vi "SimplifiedCounter.vi"() -> ()   [LabVIEW 2020]
uses:
  <vilib>/Platform/TimedLoop/XDataNode/timing_clust.ctl
  <vilib>/Platform/TimedLoop/XDataNode/nitl_modes.ctl
  <vilib>/Platform/TimedLoop/XDataNode/wakeup.ctl
  <vilib>/rvi/Emulation/niFpgaGetClockAttributes.vi
  <vilib>/rvi/Emulation/niFpgaSctlEmulationGetInTimedLoop.vi
  <vilib>/rvi/Emulation/niFpgaEmulationReportErrorSimple.vi
  <vilib>/rvi/Emulation/niFpgaCriticalErrorInLSC.vi
  <vilib>/rvi/eio/common/nirviEmuTemplateMethod_errors.vi
  <vilib>/rvi/Emulation/niFpgaProcessEmulError.vi
  <vilib>/Platform/TimedLoop/XDataNode/XDataNode.xnode
  <vilib>/eio/EIONode/EIONode.xnode
  <vilib>/Platform/TimedLoop/XDataNode/XDNodeRunTimeDep.lvlib
panel:
  out "Error":errorcluster
  out "Counter Out":i16
  in  "Reset?":bool
  in  "Count(Ticks)":u32
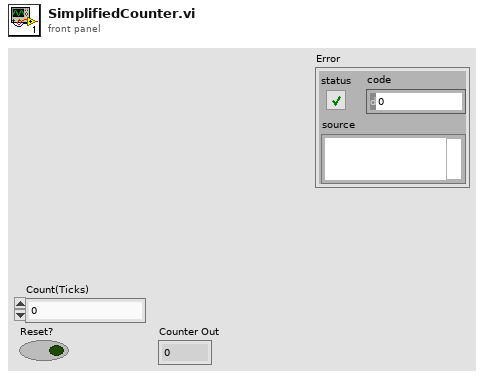
[diagram p1: front panel]
types:
  T1 = enum16{"Rising Edge", "Falling Edge", "Rising AND Falling Edges"}
  T2 = typedef "XDNodeRunTimeDep.lvlib/timing_clust.ctl" = cluster{"Expected End [f-1]":u64, "Actual End [f-1]":u64, "Finished Late? [f-1]":bool, "Expected End [i-1]":u64, "Actual End [i-1]":u64, "Finished Late? [i-1]":bool, "Expected Start [i]":u64, "Actual Start [i]":u64, "Expected Start [f]":u64, "Actual Start [f]":u64, "Source Name":string, "Structure Name":string, "Period":i64, "Deadline":i64, "Offset":i64, "Start":i64, "Priority":i32, "Timeout":i32, "Mode":T3, "Wakeup Reason":T4, "Error":errorcluster, "Source Type":string, "Secondary Source Type":string, "Global End Time":u64, "Global Start Time":u64, "Frame Duration":u64, "Iteration Duration":u64, "Assigned CPU":i32, "I/O Scan Engine Mode":u32}
  T3 = typedef "XDNodeRunTimeDep.lvlib/nitl_modes.ctl" = enum32{"No Change", "Process missed periods, maintain original phase", "Discard missed periods, maintain original phase", "Process missed periods, ignore original phase", "Discard missed periods, ignore original phase"}
  T4 = typedef "XDNodeRunTimeDep.lvlib/wakeup.ctl" = enum32{"Normal", "Aborted", "Asynchronous wakeup", "Timing source error", "Timed loop error", "Timeout"}
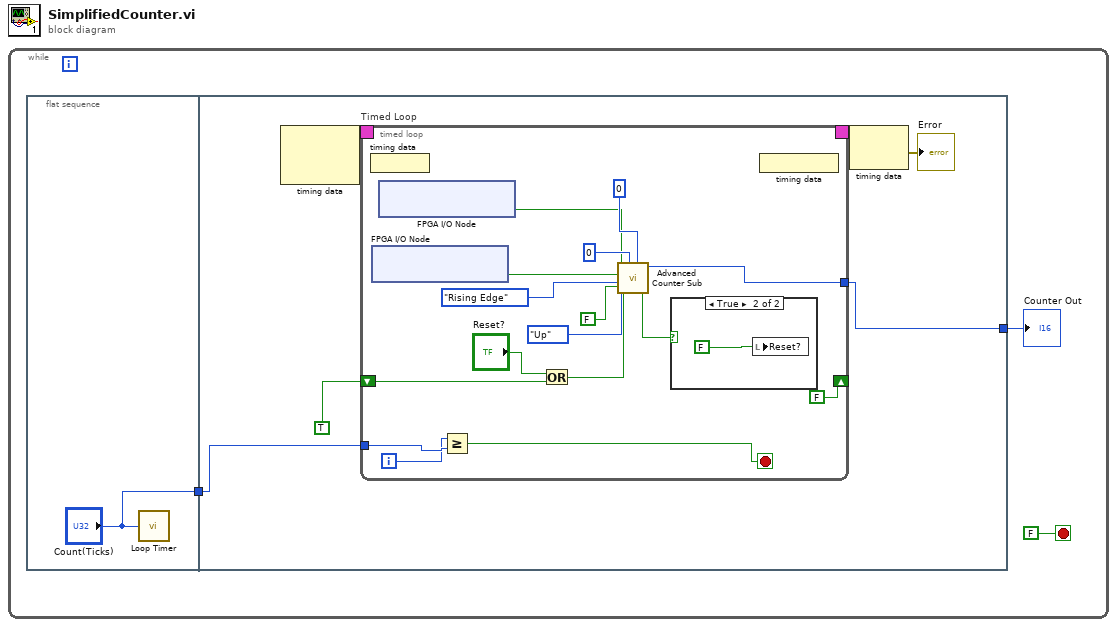
[diagram p0: block diagram]
diagram:
  n1 = while {
    stop <- FALSE stop-if-true
    n2 = flat-sequence {
      tunnel: ["Count(Ticks)"] -> w3
      tunnel: w3 -> [w7]
      tunnel: [w6] -> w2
      frame #0 {
        n3 = call "Loop Timer"("Count(Ticks)"="Count(Ticks)") -> ()  [unwired: 1 out]
      }
      frame #1 {
        n4 = node-c288() -> (w10:T2)  [unwired: 2 in]
        n5 = timed-loop "Timed Loop" {
          timing: w10 -> [_]
          timing-out: [_] -> w9
          tunnel: w7 -> [w26]
          tunnel: [w24] -> w6
          shift-right: [FALSE] -> _
          shift-left: TRUE -> [w25]
          i -> [w23]
          stop <- w12 stop-if-true
          n6 = node-c288() -> ()  [unwired: 1 in]
          n7 = xnode "FPGA I/O Node"() -> ("Connector0/DIO1"=w18:bool)  [unwired: 1 in, 1 out]
          n8 = xnode "FPGA I/O Node"() -> ("Connector0/DIO0"=w19:bool)  [unwired: 1 in, 1 out]
          n9 = Greater Or Equal?(x=w23, y=w26) -> (x >= y?=w12:bool)
          n10 = Or(x="Reset?", y=w25) -> (x .or. y?=w16:bool)
          n11 = call "Advanced Counter Sub.vi"("Reset Counter"=w16, "Init Counter Value"=i16 0, "Enable HW Gate"=FALSE, "Ticks to Filter"=i16 0, "Count Direction"=enum16{"Up", "Down"}."Up", "Edge"=T1."Rising Edge", "Gate Signal"=w18, "Input Signal"=w19) -> ("Counter Reset?"=w15:bool, "Counter Out"=w24:u32)  [unwired: 2 in]
          n12 = case shown="True" w15 {
            frame False {
            }
            frame True {
              n13 = local write "Reset?"(FALSE ("Reset?")) -> ()
            }
          }
          n14 = node-c288() -> ()  [unwired: 1 out]
        }
        n15 = node-c288(w9) -> (→"Error":errorcluster)
      }
    }
    "Counter Out" <- w2
  }
